vi "E20_Actividad_08_mayo_26.vi"   [LabVIEW 2026]
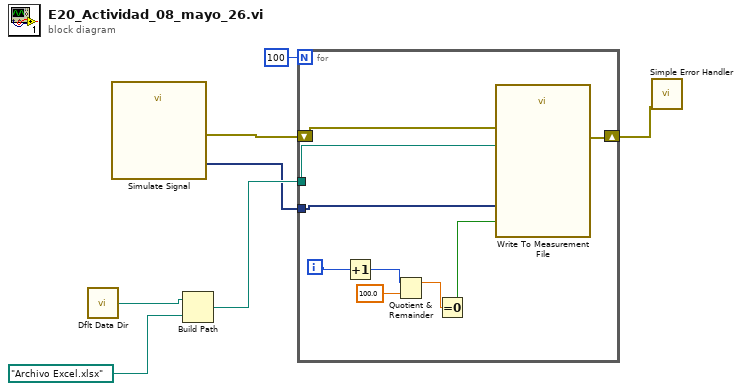
[diagram p0: block diagram]
diagram:
  n1 = call <vilib>:"Dflt Data Dir.vi"() -> ("App:Default Data Directory"=w5:path)
  n2 = call "Simulate Signal"() -> ("Sine"=w1:dynamicdata, "error out"=w6:errorcluster)  [unwired: 14 in]
  n3 = Build Path(base path=w5, name or relative path=path "Archivo Excel.xlsx") -> (appended path=w2:path)
  n4 = for {
    N: 100 -> [_]
    shift-right: [w14] -> w3
    shift-left: w6 -> [w12]
    tunnel: w2 -> [w11]
    tunnel: w1 -> [w10]
    i -> [w15]
    n5 = Increment(x=w15) -> (x+1=w8:i32)
    n6 = Quotient & Remainder(x=w8, y=100.0) -> (x-y*floor(x/y)=w9:dbl)  [unwired: 1 out]
    n7 = Equal To 0?(x=w9) -> (x = 0?=w13:bool)
    n8 = call "Write To Measurement File"("Signals"=w10, "Flush? (T)"=w13, "error in (no error)"=w12, "Filename"=w11) -> ("error out"=w14:errorcluster)  [unwired: 13 in, 2 out]
  }
  n9 = call <vilib>:"Simple Error Handler.vi"("error in (no error)"=w3) -> ()  [unwired: 4 in, 5 out]
